vi "Set Voltage.vi"(8 "error in (no error)":errorcluster, 10 "Voltage":dbl, 11 "Keysight in":refnum<class "Keysight.lvclass">) -> (0 "error out":errorcluster, 3 "Keysight out":refnum<class "Keysight.lvclass">)   [LabVIEW 2020, in "PS.lvlib" / "Keysight.lvclass"]
uses:
  Keysight.lvclass
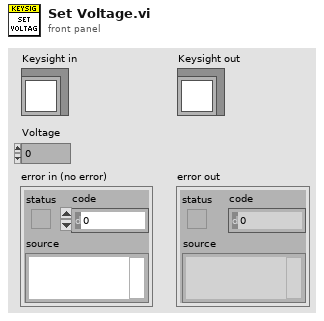
[diagram p1: front panel]
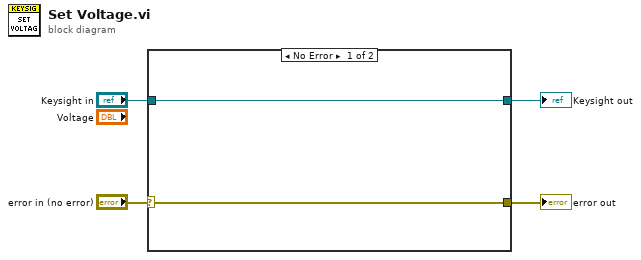
[diagram p0: block diagram]
diagram:
  n1 = case shown="No Error" "error in (no error)" {
    selector: "error in (no error)" -> [w5 w7]
    tunnel: [w6 w8] -> w3
    tunnel: "Keysight in" -> [w6 w8]
    tunnel: [w5 w7] -> w1
    frame No Error {
    }
    frame Error {
    }
  }
  "error out" <- w1
  "Keysight out" <- w3
